vi "FTW-Time-Uptime.vi"(0 "Previous Uptime":dbl format="%.3fmsec\n%<%D:%H:%M:%S%3u>t", 11 "error in":errorcluster) -> (4 "Current Uptime":dbl format="%.3fmsec\n%<%D:%H:%M:%S%3u>t", 6 "Elapsed Time":dbl format="%.6fsec", 15 "error out":errorcluster)   [LabVIEW 2013]
panel:
  # "Inputs"
  # "Outputs"
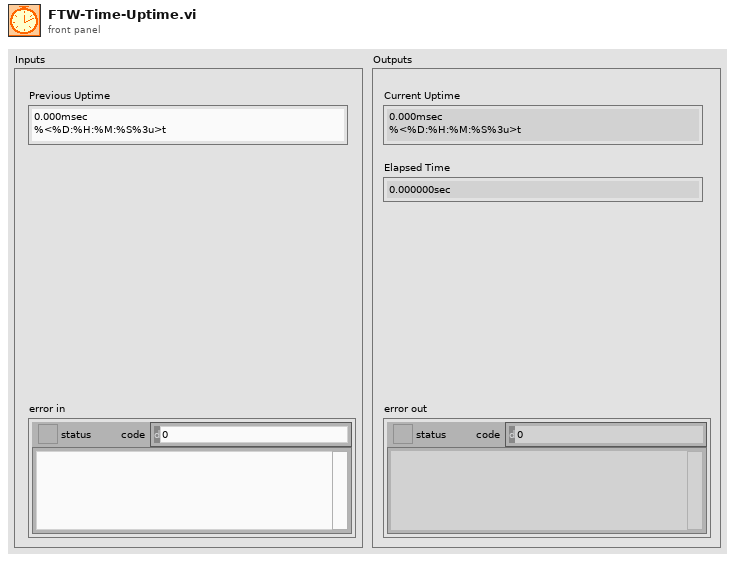
[diagram p1: front panel]
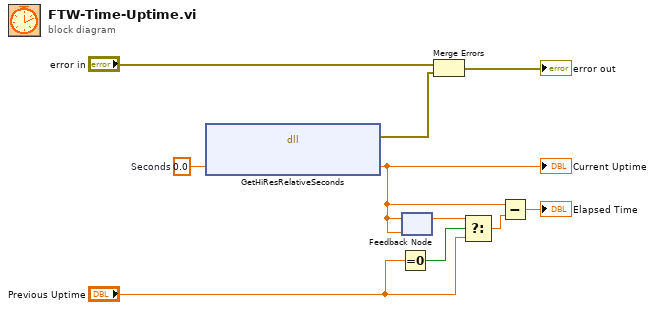
[diagram p0: block diagram]
diagram:
  w10 = 0.0  # Seconds
  n1 = dll-call lib="LabVIEW" fn="GetHiResRelativeSeconds"("Seconds"=w10) -> (error out=w1:errorcluster, "Seconds"=w5:dbl)  [unwired: 4 in, 1 out]
  "Current Uptime" <- w5
  n2 = Equal To 0?(x="Previous Uptime") -> (x = 0?=w4:bool)
  n3 = feedback-in #1(w5) -> ()
  n4 = feedback #1(w5) -> (w8:dbl)
  n5 = Merge Errors("error in", w1) -> (→"error out":errorcluster)
  n6 = Select(t=w8, s=w4, f="Previous Uptime") -> (s? t:f=w6:dbl)
  n7 = Subtract(x=w5, y=w6) -> (x-y=→"Elapsed Time":dbl)
